vi "APDM Autoconfigure.vi"(2 "error in (no error)":errorcluster, 3 "APDM Context":T1={"APDM Context ID"=0, "Gyro Mode"="", "Log Data"=FALSE, "Log File"=refnum, "Gyro Record Log"=refnum, "Gyro CMD Log"=refnum, "L Opal SN"=0, "R Opal SN"=0, "Access Point ID"=0, "Left Gyro Sim Data"=path "C:/Users/jfalesi/Desktop/CP FES Walking Code/Original/Ahad Vi/CP Code/Offline data/TD_7_Raw_R.txt", "Right Gyro Sim Data"=path "C:/Users/jfalesi/Desktop/CP FES Walking Code/Original/Ahad Vi/CP Code/Offline data/TD_7_Raw_R.txt", "Sampling Rate"=0.0, "Gyro Sim Time Array"=[], "Missed Gyro Count"=0.0}) -> (0 "error out":errorcluster, 1 "APDM Context":T1={"APDM Context ID"=0, "Gyro Mode"="", "Log Data"=FALSE, "Log File"=refnum, "Gyro Record Log"=refnum, "Gyro CMD Log"=refnum, "L Opal SN"=0, "R Opal SN"=0, "Access Point ID"=0, "Left Gyro Sim Data"=path "C:/Users/jfalesi/Desktop/CP FES Walking Code/Original/Ahad Vi/CP Code/Offline data/TD_7_Raw_R.txt", "Right Gyro Sim Data"=path "C:/Users/jfalesi/Desktop/CP FES Walking Code/Original/Ahad Vi/CP Code/Offline data/TD_7_Raw_R.txt", "Sampling Rate"=0.0, "Gyro Sim Time Array"=[], "Missed Gyro Count"=0.0})   [LabVIEW 2019]
uses:
  Controls/APDM Context Cluster.ctl
  Program Files/National Instruments/LabVIEW 2019/user.lib/apdm/apdm.lvlib
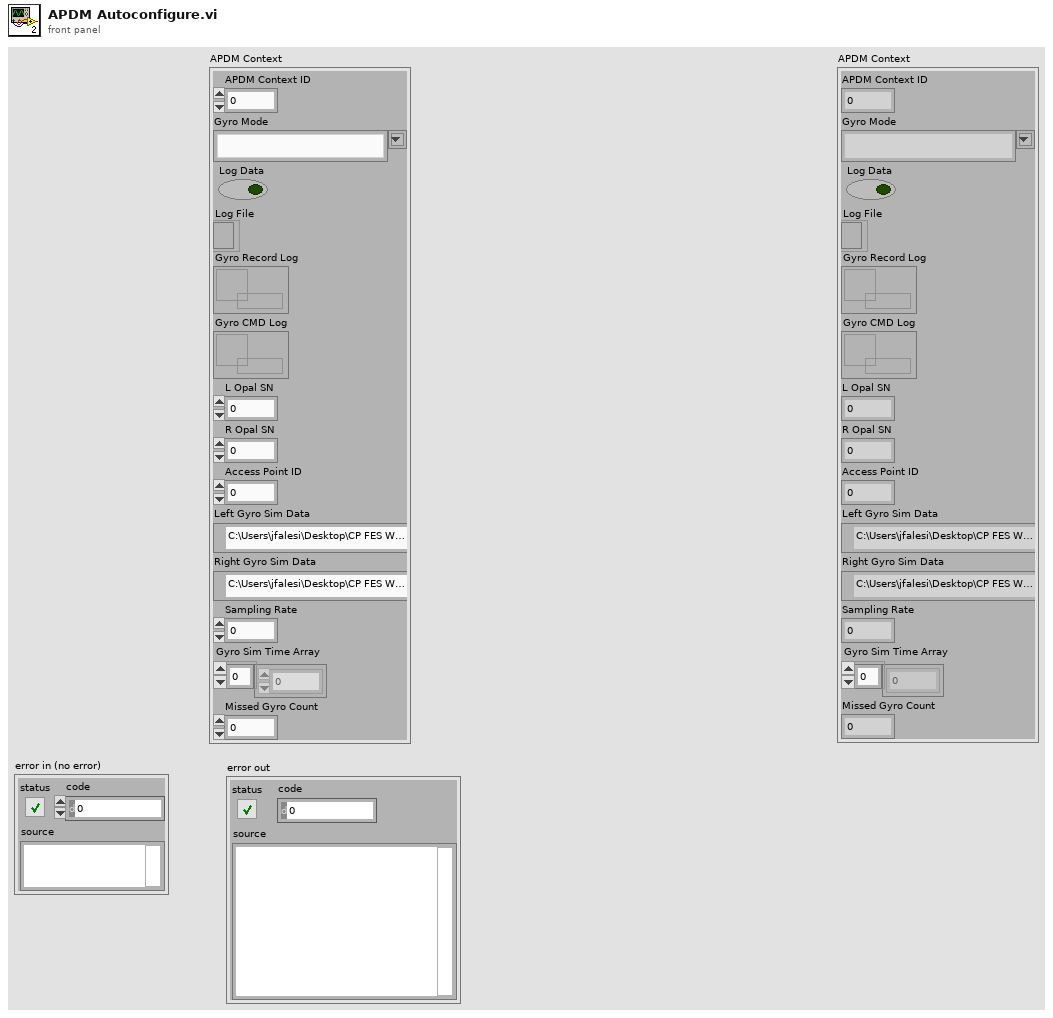
[diagram p1: front panel]
types:
  T1 = typedef "APDM Context Cluster.ctl" = cluster{"APDM Context ID":u32, "Gyro Mode":string, "Log Data":bool, "Log File":refnum<file>, "Gyro Record Log":refnum<queue>, "Gyro CMD Log":refnum<queue>, "L Opal SN":u32, "R Opal SN":u32, "Access Point ID":u32, "Left Gyro Sim Data":path, "Right Gyro Sim Data":path, "Sampling Rate":dbl, "Gyro Sim Time Array":dbl[], "Missed Gyro Count":dbl}
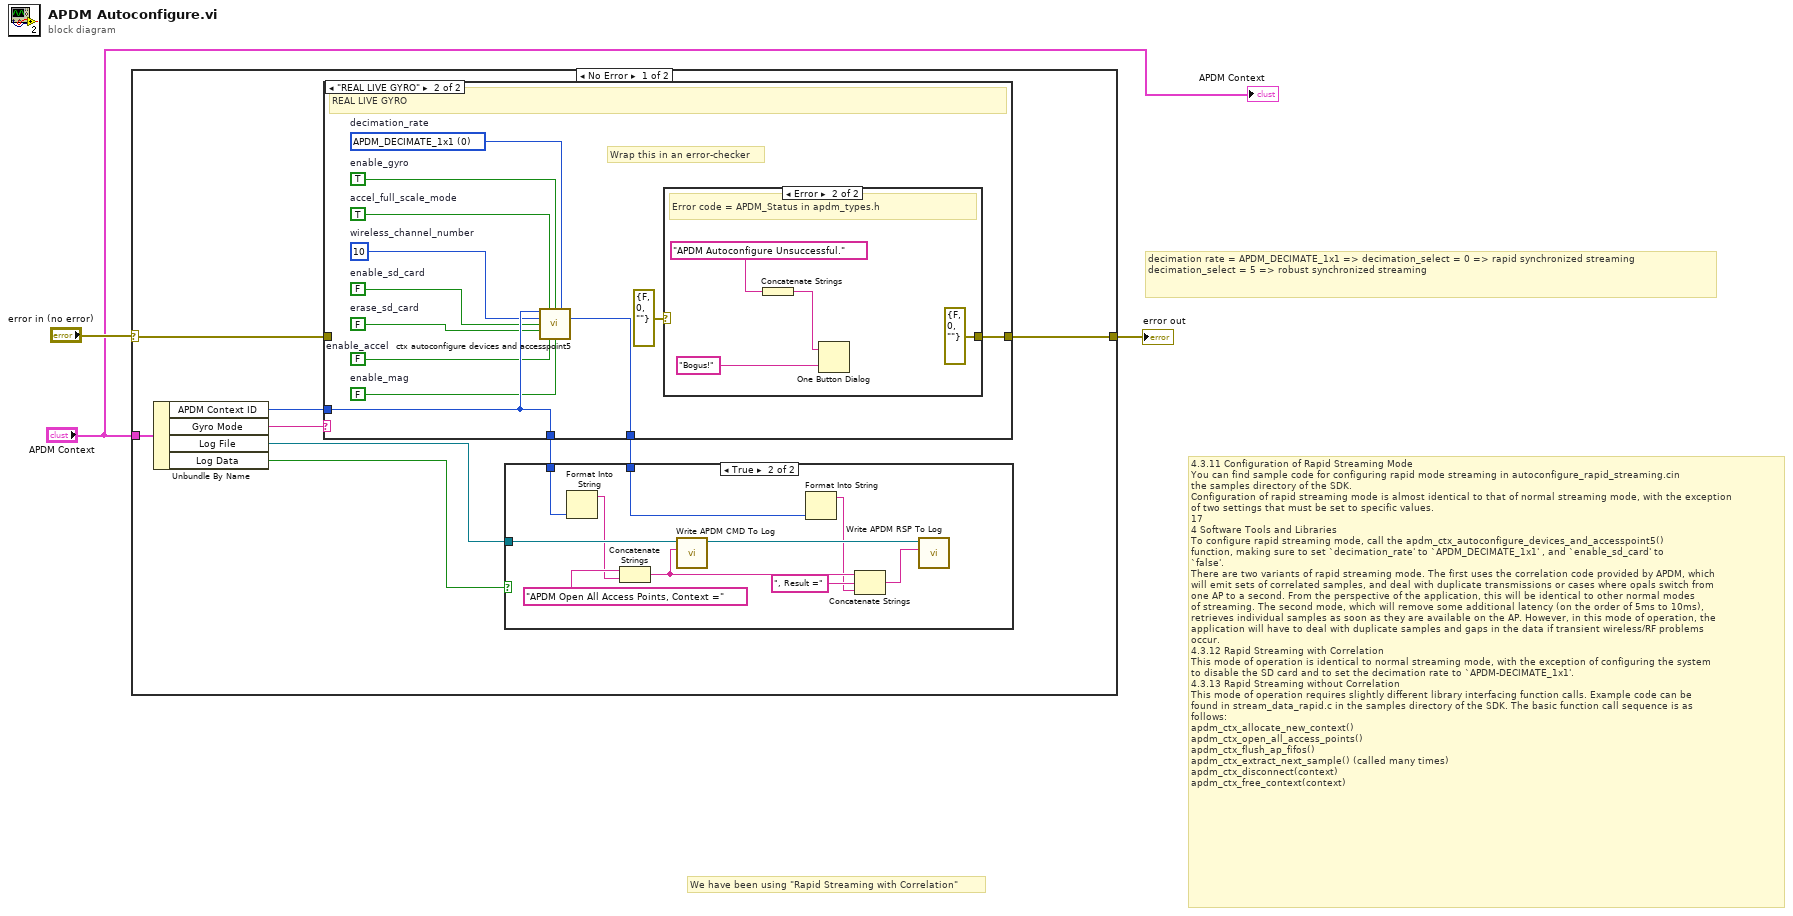
[diagram p0: block diagram]
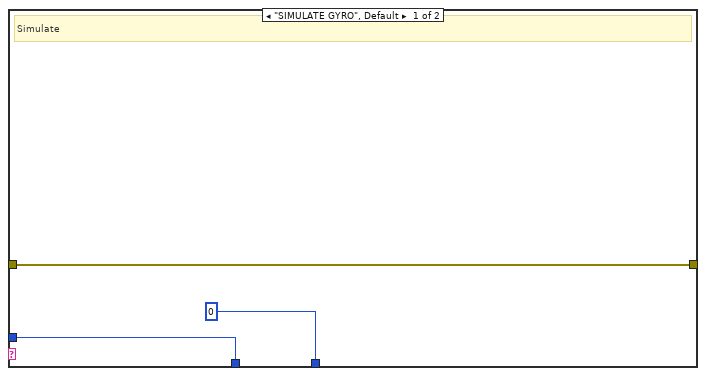
[diagram p3: hidden frame]
diagram:
  # "We have been using \"Rapid Streaming with Correlation\""
  # "4.3.11 Configuration of Rapid Streaming Mode\nYou can find sample code for configuring rapid mode streaming in autoconfigure_rapid_streaming.cin\nthe samples directory of the SDK.\nConfiguration of rapid streaming mode is almost identical to that of normal streaming mode, with the exception\nof two settings that must be set to specific values.\n17\n4 Software Tools and Libraries\nTo configure rapid streaming mode, call the apdm_ctx_autoconfigure_devices_and_accesspoint5()\nfunction, making sure to set `decimation_rate' to `APDM_DECIMATE_1x1' , and `enable_sd_card' to\n`false'.\nThere are two variants of rapid streaming mode. The first uses the correlation code provided by APDM, which\nwill emit sets of correlated samples, and deal with duplicate transmissions or cases where opals switch from\none AP to a second. From the perspective of the application, this will be identical to other normal modes\nof streaming. The second mode, which will remove some additional latency (on the order of 5ms to 10ms),\nretrieves individual samples as soon as they are available on the AP. However, in this mode of operation, the\napplication will have to deal with duplicate samples and gaps in the data if transient wireless/RF problems\noccur.\n4.3.12 Rapid Streaming with Correlation\nThis mode of operation is identical to normal streaming mode, with the exception of configuring the system\nto disable the SD card and to set the decimation rate to `APDM-DECIMATE_1x1'.\n4.3.13 Rapid Streaming without Correlation\nThis mode of operation requires slightly different library interfacing function calls. Example code can be\nfound in stream_data_rapid.c in the samples directory of the SDK. The basic function call sequence is as\nfollows:\napdm_ctx_allocate_new_context()\napdm_ctx_open_all_access_points()\napdm_ctx_flush_ap_fifos()\napdm_ctx_extract_next_sample() (called many times)\napdm_ctx_disconnect(context)\napdm_ctx_free_context(context)"
  # "decimation rate = APDM_DECIMATE_1x1 => decimation_select = 0 => rapid synchronized streaming\ndecimation_select = 5 => robust synchronized streaming"
  n1 = case shown="No Error" "error in (no error)" {
    selector: "error in (no error)" -> [w5 w43]
    tunnel: [w12 w43] -> w3
    tunnel: "APDM Context" -> [w4 _]
    frame No Error {
      n2 = Unbundle By Name(w4) -> ("APDM Context ID"=w10:u32, "Gyro Mode"=w9:string, "Log File"=w7:refnum<file>, "Log Data"=w8:bool)
      n3 = case shown="\"REAL LIVE GYRO\"" w9 {
        tunnel: w10 -> [w23 w37]
        tunnel: [w25 w26] -> w12
        tunnel: w5 -> [w25 _]
        tunnel: [0 w28] -> w11
        tunnel: [w23 w37] -> w6
        frame "SIMULATE GYRO", Default {
          # "Simulate"
        }
        frame "REAL LIVE GYRO" {
          w29 = FALSE  # enable_mag
          w30 = FALSE  # enable_accel
          w31 = FALSE  # erase_sd_card
          w32 = FALSE  # enable_sd_card
          w33 = u32 0 items=["APDM_DECIMATE_1x1", "APDM_DECIMATE_2x1", "APDM_DECIMATE_2x2", "APDM_DECIMATE_5x1", "APDM_DECIMATE_4x2", "APDM_DECIMATE_5x2", "APDM_DECIMATE_4x4", "APDM_DECIMATE_5x4", "APDM_DECIMATE_8x4", "APDM_DECIMATE_8x5", "APDM_DECIMATE_8x8"]  # decimation_rate
          w34 = TRUE  # enable_gyro
          w35 = TRUE  # accel_full_scale_mode
          w36 = u8 10  # wireless_channel_number
          # "Wrap this in an error-checker"
          # "REAL LIVE GYRO"
          n4 = call "ctx autoconfigure devices and accesspoint5.vi"("context"=w37, "accel_full_scale_mode"=w35, "enable_gyro"=w34, "decimation_rate"=w33, "wireless_channel_number"=w36, "enable_sd_card"=w32, "erase_sd_card"=w31, "enable_accel"=w30, "enable_mag"=w29) -> ("function return"=w28:i32)  [unwired: 5 in, 1 out]
          n5 = case shown="Error" errorcluster {"status"=FALSE, "code"=0, "source"=""} ("error IO") {
            selector: errorcluster {"status"=FALSE, "code"=0, "source"=""} ("error IO") -> [w38 _]
            tunnel: [w38 errorcluster {"status"=FALSE, "code"=0, "source"=""} ("error IO")] -> w26
            frame No Error {
              # "Success"
            }
            frame Error {
              # "Error code = APDM_Status in apdm_types.h"
              n6 = Concatenate Strings("APDM Autoconfigure Unsuccessful." ("string")) -> (w40:string)
              n7 = One Button Dialog(message=w40, button name ("OK")="Bogus!") -> ()  [unwired: 1 out]
            }
          }
        }
      }
      n8 = case shown="True" w8 {
        tunnel: w11 -> [_ w21]
        tunnel: w7 -> [_ w20]
        tunnel: w6 -> [_ w18]
        frame False {
        }
        frame True {
          n9 = Format Into String(w18) -> (resulting string=w17:string)  [unwired: 3 in, 1 out]
          n10 = Concatenate Strings("APDM Open All Access Points, Context =" ("Log Item"), w17) -> (w16:string)
          n11 = call "Write APDM CMD To Log.vi"("Log Item"=w16, "Byte Stream File in"=w20) -> ("Byte Stream File out"=w22:refnum<file>)  [unwired: 8 in, 1 out]
          n12 = Format Into String(w21) -> (resulting string=w14:string)  [unwired: 3 in, 1 out]
          n13 = Concatenate Strings(w16, ", Result =" ("Log Item"), w14) -> (w13:string)
          n14 = call "Write APDM RSP To Log.vi"("Log Item"=w13, "Byte Stream File in"=w22) -> ()  [unwired: 9 in, 1 out]
        }
      }
    }
    frame Error {
    }
  }
  "error out" <- w3
  "APDM Context" <- "APDM Context"
